vi "限幅器（SGL）.vi"(3 "下限":sgl, 4 "X_in":sgl, 5 "上限":sgl) -> (1 "X_Out":sgl)   [LabVIEW 2012]
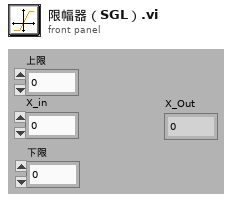
[diagram p1: front panel]
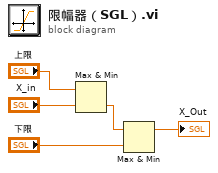
[diagram p0: block diagram]
diagram:
  n1 = Max & Min(x="上限", y="X_in") -> (min(x,y)=w3:sgl)  [unwired: 1 out]
  n2 = Max & Min(x=w3, y="下限") -> (max(x,y)=→"X_Out":sgl)  [unwired: 1 out]
